vi "Count.vi"(3 "MsgPackArray in":refnum<class "MsgPackArray.lvclass">) -> (1 "Count":u64)   [LabVIEW 2020, in "MessagePack.lvlib" / "MsgPackArray.lvclass"]
uses:
  MsgPackArray.lvclass
  MsgPackArray.lvclass/MsgPackArray.ctl
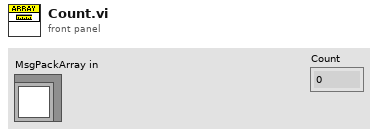
[diagram p1: front panel]
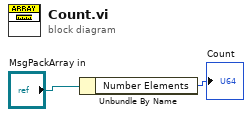
[diagram p0: block diagram]
diagram:
  n1 = Unbundle By Name("MsgPackArray in") -> ("Number Elements"=→"Count":u32)
